vi "7SegmentMod2.vi"() -> ()   [LabVIEW 2014]
doc: "\"Discrete LED demo.vi\" -- Demonstrate a discrete LED connected to a digital output.\n\nInstructions:\n\n-- Click the 'enable blinker' button to toggle between blinking mode\nand static mode.\n-- In static mode, click the 'digital level' button to set the state of the\ndigital output.\n-- The 'digital output state' LED indicator shows the state of the\ndigital output (on = high, off = low)."
uses:
  <vilib>/myRIO/Instrument Drivers/Onboard IO/DIO/vis/Write.vi
  <vilib>/myRIO/Common/Instrument Driver Framework/myRIO v1.0/UART/vis/myRIO v1.0 Close UART.vi
  <vilib>/myRIO/Instrument Drivers/Onboard IO/DIO/vis/Smart Open.vi
  <vilib>/Utility/error.llb/Error Cluster From Error Code.vi
  <vilib>/myRIO/Common/Instrument Driver Framework/myRIO v1.0/DIO/vis/myRIO v1.0 Write DIO.vi
  <vilib>/myRIO/Common/Instrument Driver Framework/Utilities/vis/FPGA Ref Manager.vi
  <vilib>/myRIO/Common/Instrument Driver Framework/myRIO v1.0/myRIO v1.0 Reset FPGA.vi
  <vilib>/myRIO/Common/Instrument Driver Framework/myRIO v1.0/IRQ/vis/myRIO v1.0 IRQ Info FGV.vi
  <vilib>/myRIO/Common/Instrument Driver Framework/myRIO v1.0/IRQ/vis/myRIO v1.0 Timer IRQ Info FGV.vi
  <vilib>/myRIO/Common/Instrument Driver Framework/myRIO v1.0/IRQ/vis/myRIO v1.0 ISR Agent.vi
  <vilib>/myRIO/Instrument Drivers/Utilities/Utilities.lvlib
panel:
  in  "Control":T1(ring)
  in  "[ESC]":bool
  # "7-Segment LED demo"
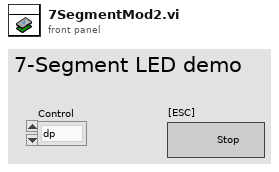
[diagram p1: front panel]
types:
  T1 = enum16{"dp", "9", "8", "7", "6", "5", "4", "3", "2", "1", "0"}
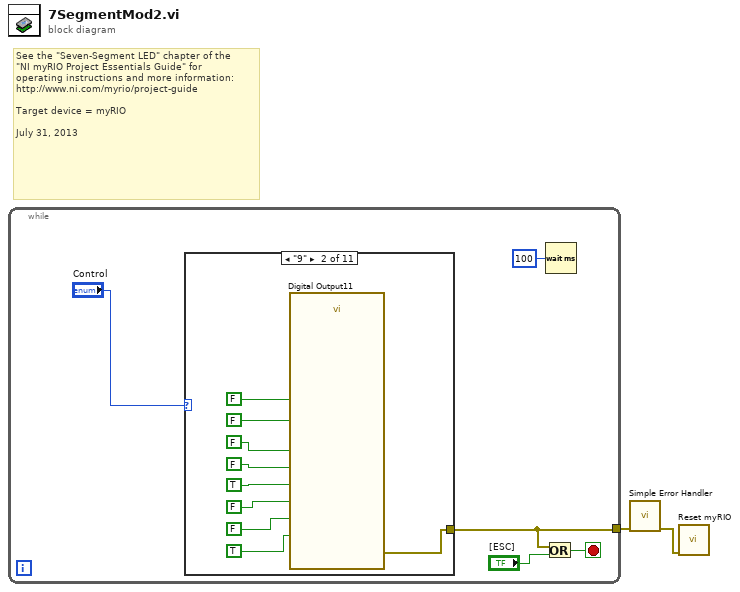
[diagram p0: block diagram]
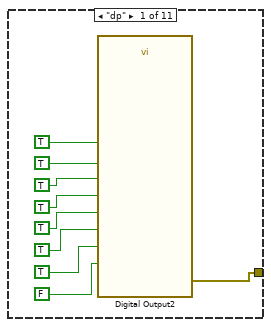
[diagram p2: hidden frame]
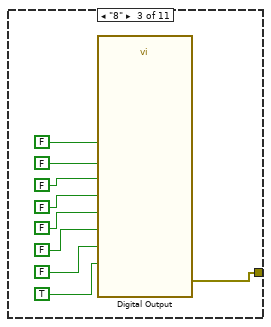
[diagram p3: hidden frame]
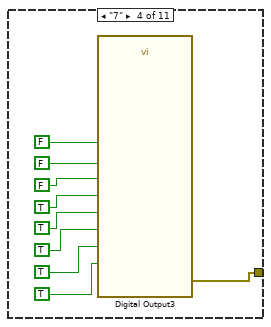
[diagram p4: hidden frame]
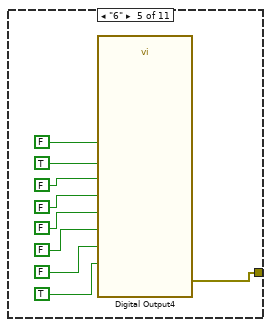
[diagram p5: hidden frame]
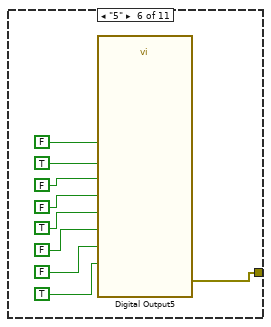
[diagram p6: hidden frame]
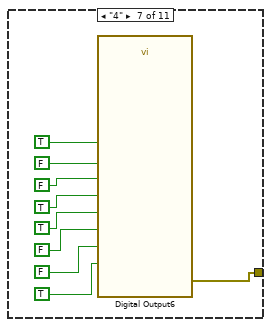
[diagram p7: hidden frame]
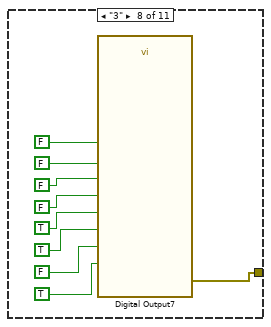
[diagram p8: hidden frame]
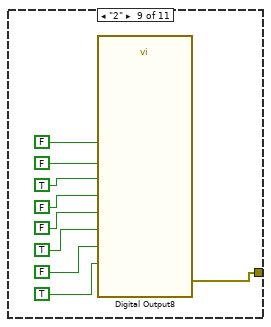
[diagram p9: hidden frame]
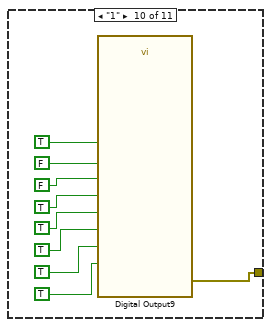
[diagram p10: hidden frame]
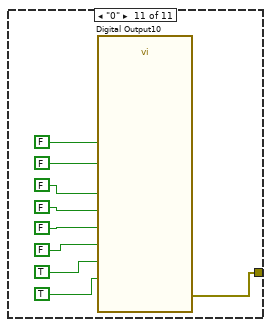
[diagram p11: hidden frame]
diagram:
  # "See the \"Seven-Segment LED\" chapter of the\n\"NI myRIO Project Essentials Guide\" for\noperating instructions and more information: \nhttp://www.ni.com/myrio/project-guide\n\nTarget device = myRIO\n\nJuly 31, 2013"
  n1 = while {
    tunnel: [w5] -> w2
    stop <- w7 stop-if-true
    n2 = case shown="\"9\"" "Control" {
      tunnel: [w16 w25 w34 w43 w52 w61 w70 w79 w88 w97 w106] -> w5
      frame "dp" {
        n3 = call "Digital Output2"("B/DIO0 (Pin 11)"=TRUE, "B/DIO1 (Pin 13)"=TRUE, "B/DIO2 (Pin 15)"=TRUE, "B/DIO3 (Pin 17)"=TRUE, "B/DIO4 (Pin 19)"=TRUE, "B/DIO5 (Pin 21)"=TRUE, "B/DIO6 (Pin 23)"=TRUE, "B/DIO7 (Pin 25)"=FALSE) -> ("error out"=w16:errorcluster)  [unwired: 19 in]
      }
      frame "9" {
        n4 = call "Digital Output11"("B/DIO0 (Pin 11)"=FALSE, "B/DIO1 (Pin 13)"=FALSE, "B/DIO2 (Pin 15)"=FALSE, "B/DIO3 (Pin 17)"=FALSE, "B/DIO4 (Pin 19)"=TRUE, "B/DIO5 (Pin 21)"=FALSE, "B/DIO6 (Pin 23)"=FALSE, "B/DIO7 (Pin 25)"=TRUE) -> ("error out"=w25:errorcluster)  [unwired: 19 in]
      }
      frame "8" {
        n5 = call "Digital Output"("B/DIO0 (Pin 11)"=FALSE, "B/DIO1 (Pin 13)"=FALSE, "B/DIO2 (Pin 15)"=FALSE, "B/DIO3 (Pin 17)"=FALSE, "B/DIO4 (Pin 19)"=FALSE, "B/DIO5 (Pin 21)"=FALSE, "B/DIO6 (Pin 23)"=FALSE, "B/DIO7 (Pin 25)"=TRUE) -> ("error out"=w34:errorcluster)  [unwired: 19 in]
      }
      frame "7" {
        n6 = call "Digital Output3"("B/DIO0 (Pin 11)"=FALSE, "B/DIO1 (Pin 13)"=FALSE, "B/DIO2 (Pin 15)"=FALSE, "B/DIO3 (Pin 17)"=TRUE, "B/DIO4 (Pin 19)"=TRUE, "B/DIO5 (Pin 21)"=TRUE, "B/DIO6 (Pin 23)"=TRUE, "B/DIO7 (Pin 25)"=TRUE) -> ("error out"=w43:errorcluster)  [unwired: 19 in]
      }
      frame "6" {
        n7 = call "Digital Output4"("B/DIO0 (Pin 11)"=FALSE, "B/DIO1 (Pin 13)"=TRUE, "B/DIO2 (Pin 15)"=FALSE, "B/DIO3 (Pin 17)"=FALSE, "B/DIO4 (Pin 19)"=FALSE, "B/DIO5 (Pin 21)"=FALSE, "B/DIO6 (Pin 23)"=FALSE, "B/DIO7 (Pin 25)"=TRUE) -> ("error out"=w52:errorcluster)  [unwired: 19 in]
      }
      frame "5" {
        n8 = call "Digital Output5"("B/DIO0 (Pin 11)"=FALSE, "B/DIO1 (Pin 13)"=TRUE, "B/DIO2 (Pin 15)"=FALSE, "B/DIO3 (Pin 17)"=FALSE, "B/DIO4 (Pin 19)"=TRUE, "B/DIO5 (Pin 21)"=FALSE, "B/DIO6 (Pin 23)"=FALSE, "B/DIO7 (Pin 25)"=TRUE) -> ("error out"=w61:errorcluster)  [unwired: 19 in]
      }
      frame "4" {
        n9 = call "Digital Output6"("B/DIO0 (Pin 11)"=TRUE, "B/DIO1 (Pin 13)"=FALSE, "B/DIO2 (Pin 15)"=FALSE, "B/DIO3 (Pin 17)"=TRUE, "B/DIO4 (Pin 19)"=TRUE, "B/DIO5 (Pin 21)"=FALSE, "B/DIO6 (Pin 23)"=FALSE, "B/DIO7 (Pin 25)"=TRUE) -> ("error out"=w70:errorcluster)  [unwired: 19 in]
      }
      frame "3" {
        n10 = call "Digital Output7"("B/DIO0 (Pin 11)"=FALSE, "B/DIO1 (Pin 13)"=FALSE, "B/DIO2 (Pin 15)"=FALSE, "B/DIO3 (Pin 17)"=FALSE, "B/DIO4 (Pin 19)"=TRUE, "B/DIO5 (Pin 21)"=TRUE, "B/DIO6 (Pin 23)"=FALSE, "B/DIO7 (Pin 25)"=TRUE) -> ("error out"=w79:errorcluster)  [unwired: 19 in]
      }
      frame "2" {
        n11 = call "Digital Output8"("B/DIO0 (Pin 11)"=FALSE, "B/DIO1 (Pin 13)"=FALSE, "B/DIO2 (Pin 15)"=TRUE, "B/DIO3 (Pin 17)"=FALSE, "B/DIO4 (Pin 19)"=FALSE, "B/DIO5 (Pin 21)"=TRUE, "B/DIO6 (Pin 23)"=FALSE, "B/DIO7 (Pin 25)"=TRUE) -> ("error out"=w88:errorcluster)  [unwired: 19 in]
      }
      frame "1" {
        n12 = call "Digital Output9"("B/DIO0 (Pin 11)"=TRUE, "B/DIO1 (Pin 13)"=FALSE, "B/DIO2 (Pin 15)"=FALSE, "B/DIO3 (Pin 17)"=TRUE, "B/DIO4 (Pin 19)"=TRUE, "B/DIO5 (Pin 21)"=TRUE, "B/DIO6 (Pin 23)"=TRUE, "B/DIO7 (Pin 25)"=TRUE) -> ("error out"=w97:errorcluster)  [unwired: 19 in]
      }
      frame "0" {
        n13 = call "Digital Output10"("B/DIO0 (Pin 11)"=FALSE, "B/DIO1 (Pin 13)"=FALSE, "B/DIO2 (Pin 15)"=FALSE, "B/DIO3 (Pin 17)"=FALSE, "B/DIO4 (Pin 19)"=FALSE, "B/DIO5 (Pin 21)"=FALSE, "B/DIO6 (Pin 23)"=TRUE, "B/DIO7 (Pin 25)"=TRUE) -> ("error out"=w106:errorcluster)  [unwired: 19 in]
      }
    }
    n14 = Or(x=w5, y="[ESC]") -> (x .or. y?=w7:bool)
    n15 = Wait (ms)(milliseconds to wait=u32 100) -> ()  [unwired: 1 out]
  }
  n16 = call <vilib>:"Simple Error Handler.vi"("error in (no error)"=w2) -> ("error out"=w1:errorcluster)  [unwired: 4 in, 4 out]
  n17 = call <vilib>:"Reset myRIO.vi"("error in (no error)"=w1) -> ()  [unwired: 10 in, 1 out]
